vi "Check for Holding Register Mapping Conflicts.vi"(8 "error in (no error)":errorcluster, 11 "Group Ref in":T1 format="%.0x") -> (0 "error out":errorcluster, 1 "Conflicts?":bool, 2 "Conflicts":T2(array[cluster]), 3 "Coil Group Ref out":T1 format="%.0x")   [LabVIEW 2020, in "Modbus Master System Explorer.lvlib"]
uses:
  Modbus Master System Explorer.lvlib
  <vilib>/NI VeriStand/Custom Device API/Custom Device Item Ref.ctl
  Modbus Type.ctl
  <vilib>/NI VeriStand/Custom Device API/Custom Device API.lvlib
  Shared/Modbus Master Shared.lvlib
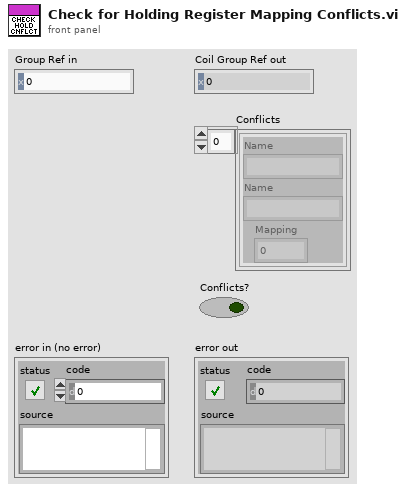
[diagram p1: front panel]
types:
  T1 = typedef "Custom Device API.lvlib/Custom Device Item Ref.ctl" = u64
  T2 = cluster{"Name":string, "Name":string, "Mapping":u16}[]
  T3 = typedef "Modbus Master Shared.lvlib/Modbus Type.ctl" = enum16{"Coil", "Discrete Input", "Holding Register", "Input Register"}
  T4 = typedef "Modbus Master Shared.lvlib/Mapping.ctl" = cluster{"DataType":T5, "Starting Address":u16, "Sub-Index (Bool)":u16, "VS Reference":T1}
  T5 = typedef "Modbus Master Shared.lvlib/DataType.ctl" = enum16{"Double", "Single", "I64", "I32", "I16", "I8", "U64", "U32", "U16", "U8", "Boolean"}
  T6 = typedef "Custom Device API.lvlib/Custom Device Item Info.ctl" = cluster{"Name":string, "Is Channel":bool, "GUID":string, "Is Waveform":bool}
  T7 = cluster{"Name":string, "Name":string, "Mapping":u16}
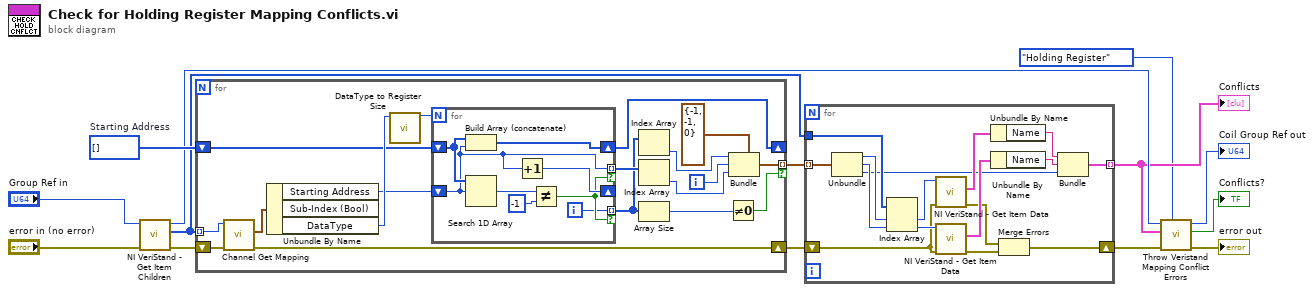
[diagram p0: block diagram]
diagram:
  w14 = u16[] []  # Starting Address
  n1 = call <vilib>:"NI VeriStand - Get Item Children.vi"("error in (no error)"="error in (no error)", "Item Ref in"="Group Ref in") -> ("error out"=w3:errorcluster, "Child Refs"=w4:T1[], "Item Ref out"=w10:T1)  [unwired: 6 in, 1 out]
  n2 = for {
    shift-right: [w25] -> _
    shift-left: w14 -> [w26]
    tunnel: [w31] -> w2 mode=indexing if=w23
    tunnel: w4 -> [w17] mode=indexing
    shift-right: [w15] -> w1
    shift-left: w3 -> [w16]
    i -> [w30]
    n3 = call "Channel Get Mapping.vi"("error in (no error)"=w16, "Item Ref in"=w17) -> ("error out"=w15:errorcluster, "Mapping"=w18:T4)  [unwired: 7 in, 1 out]
    n4 = Unbundle By Name(w18) -> ("Starting Address"=w27:u16, "DataType"=w29:T5)  [unwired: 1 out]
    n5 = call "DataType to Register Size.vi"("DataType"=w29) -> ("Registers"=w28:i32)  [unwired: 9 in, 1 out]
    n6 = for {
      N: w28 -> [_]
      shift-right: [w38] -> w25
      shift-left: w26 -> [w40]
      shift-right: [w39] -> _
      shift-left: w27 -> [w35]
      tunnel: [w33] -> w20 mode=indexing if=w34
      tunnel: [w35] -> w22 mode=indexing if=w34
      i -> [w33]
      n7 = Build Array (concatenate)(w40, w35) -> (w38:u16[])
      n8 = Search 1D Array(1D array=w40, element=w35) -> (index of element=w36:i32)  [unwired: 1 in]
      n9 = Increment(x=w35) -> (x+1=w39:u16)
      n10 = Not Equal?(x=w36, y=-1) -> (x != y?=w34:bool)
    }
    n11 = Index Array(array=w20) -> (element=w19:i32)  [unwired: 1 in]
    n12 = Index Array(array=w22) -> (element=w21:u16)  [unwired: 1 in]
    n13 = Array Size(array=w20) -> (size(s)=w24:i32)
    n14 = Not Equal To 0?(x=w24) -> (x != 0?=w23:bool)
    n15 = Bundle(cluster=cluster{"y":i32, "y 2":i32, "Mapping":u16} {"y"=-1, "y 2"=-1, "Mapping"=0} ("Conflicting Indices"), "y"=w19, "y 2"=w30, "Mapping"=w21) -> (w31:cluster{"y":i32, "y 2":i32, "Mapping":u16})
  }
  n16 = for {
    tunnel: w2 -> [w56] mode=indexing
    tunnel: w4 -> [w55]
    tunnel: [w46] -> w9 mode=indexing
    shift-right: [w41] -> w8
    shift-left: w1 -> [w44]
    n17 = Unbundle(w56) -> ("y"=w54:i32, "y 2"=w53:i32, "Mapping"=w45:u16)
    n18 = Index Array(array=w55, index #1=w54, index #2=w53) -> (element #1=w52:T1, element #2=w51:T1)
    n19 = call <vilib>:"NI VeriStand - Get Item Data.vi"("error in (no error)"=w44, "Item Ref in"=w52) -> ("error out"=w43:errorcluster, "Item Info"=w50:T6)  [unwired: 8 out]
    n20 = call <vilib>:"NI VeriStand - Get Item Data.vi"("error in (no error)"=w44, "Item Ref in"=w51) -> ("error out"=w42:errorcluster, "Item Info"=w49:T6)  [unwired: 8 out]
    n21 = Unbundle By Name(w50) -> ("Name"=w48:string)
    n22 = Unbundle By Name(w49) -> ("Name"=w47:string)
    n23 = Merge Errors(w43, w42) -> (w41:errorcluster)
    n24 = Bundle("Name"=w48, "Name"=w47, "Mapping"=w45) -> (w46:T7)  [unwired: 1 in]
  }
  "Conflicts" <- w9
  n25 = call "Throw Veristand Mapping Conflict Errors.vi"("Type"=Modbus_Type."Holding Register", "error in (no error)"=w8, "Conflicts In"=w9, "Item Ref in"=w10) -> ("error out"=→"error out":errorcluster, "Conflicts?"=→"Conflicts?":bool, "Node Ref out"=→"Coil Group Ref out":T1)  [unwired: 5 in]
